vi "tmp_toml_dump.vi"(4 "vi":refnum<vi>, 8 "error in (no error)":errorcluster, 10 "operation (replace or create)":T1(ring)=enum."replace or create", 11 "path in":path) -> (0 "error out":errorcluster, 2 "file exists":bool, 3 "path out":path)   [LabVIEW 2017]
uses:
  <vilib>/Utility/error.llb/Clear Errors.vi
  <vilib>/Utility/file.llb/Application Directory.vi
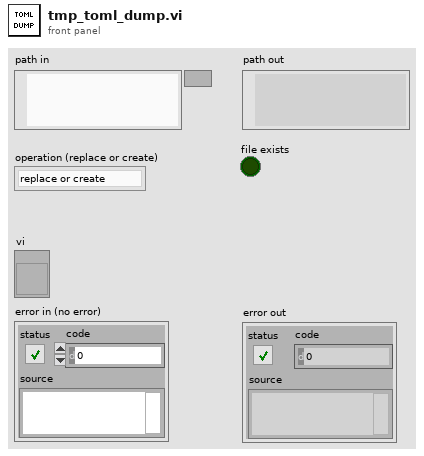
[diagram p1: front panel]
types:
  T1 = enum16{"open", "replace", "create", "open or create", "replace or create", "replace or create with confirmation"}
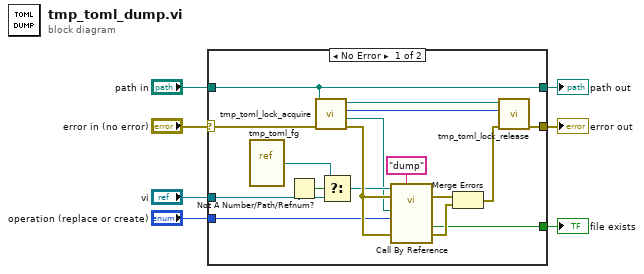
[diagram p0: block diagram]
diagram:
  n1 = case shown="No Error" "error in (no error)" {
    selector: "error in (no error)" -> [w22 w25]
    tunnel: [w18 w25] -> w6
    tunnel: "vi" -> [w15 _]
    tunnel: "path in" -> [w12 w26]
    tunnel: [w12 w26] -> w3
    tunnel: [w9 _] -> w2
    tunnel: "operation (replace or create)" -> [w8 _]
    frame No Error {
      n2 = vi-ref "tmp_toml_fg.vi"() -> (w14:refnum<vi>)
      n3 = Not A Number/Path/Refnum?(number/path/refnum=w15) -> (NaN/Path/Refnum?=w16:bool)
      n4 = call "tmp_toml_lock_acquire.vi"("error in (no error)"=w22, "path in"=w12) -> ("error out"=w21:errorcluster, "resolved path"=w11:path, "cnt"=w23:u8, "lock"=w24:refnum<queue>)  [unwired: 6 in]
      n5 = Select(t=w14, s=w16, f=w15) -> (s? t:f=w13:refnum<vi>)
      n6 = call-by-ref "?"(reference=w13, error in=w21, "cmd"="dump", 8:"error in (no error)"=w21, "data in"=w8, "path in"=w11) -> (error out=w20:errorcluster, 0:"error out"=w10:errorcluster, "return"=w9:bool)  [unwired: 4 in, 3 out]
      n7 = Merge Errors(w20, w10) -> (w19:errorcluster)
      n8 = call "tmp_toml_lock_release.vi"("error in (no error)"=w19, "cnt"=w23, "lock"=w24) -> ("error out"=w18:errorcluster)  [unwired: 8 in]
    }
    frame Error {
    }
  }
  "error out" <- w6
  "path out" <- w3
  "file exists" <- w2
